vi "Actor Receive.vi"(11 "Self Actor in":refnum<class "Self Actor.lvclass">) -> (2 "Msg":refnum<class "Msg Strategy.lvclass">, 3 "Self Actor out":refnum<class "Self Actor.lvclass">)   [LabVIEW 2021, in "jettl.lvlib" / "Self Actor.lvclass"]
uses:
  Self Actor.lvclass
  Msg Strategy/Msg Strategy.lvclass
  Self Actor.lvclass/Self Actor.ctl
  Self Actor State/Self Actor State.lvclass
  jettl.lvlib
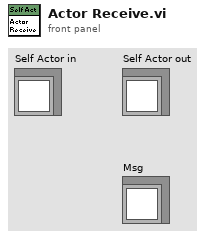
[diagram p1: front panel]
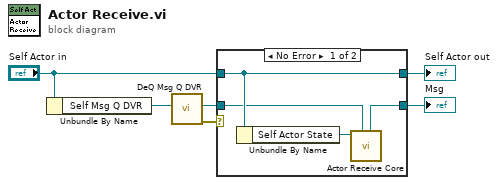
[diagram p0: block diagram]
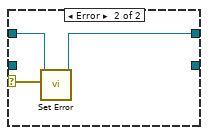
[diagram p2: hidden frame]
diagram:
  n1 = Unbundle By Name("Self Actor in") -> ("Self Msg Q DVR"=w6:refnum<data-value>)
  n2 = call "DeQ Msg Q DVR.vi"("Msg Q DVR"=w6) -> ("error out"=w5:errorcluster, "Msg"=w3:refnum<class "Msg Strategy.lvclass">)  [unwired: 9 in]
  n3 = case shown="No Error" w5 {
    selector: w5 -> [_ w11]
    tunnel: [w7 _] -> w4
    tunnel: w3 -> [w8 _]
    tunnel: "Self Actor in" -> [w9 w13]
    tunnel: [w9 w12] -> w1
    frame No Error {
      n4 = Unbundle By Name(w9) -> ("Self Actor State"=w10:refnum<class "Self Actor State.lvclass">)
      n5 = call-dynamic "Actor Receive Core.vi"("Msg in"=w8, "Self Actor State in"=w10) -> ("Msg out"=w7:refnum<class "Msg Strategy.lvclass">)  [unwired: 9 in]
    }
    frame Error {
      n6 = call-dynamic "Set Error.vi"("Error"=w11, "Self Actor in"=w13) -> ("Self Actor out"=w12:refnum<class "Self Actor.lvclass">)  [unwired: 9 in]
    }
  }
  "Msg" <- w4
  "Self Actor out" <- w1
